vi "popularVideos.vi"(8 "error in (no error)":errorcluster, 11 "ThirdPartyYoutubeLib in":refnum<class "ThirdPartyYoutubeLib.lvclass">) -> (0 "error out":errorcluster, 2 "HashMap":T1, 3 "ThirdPartyYoutubeLib out":refnum<class "ThirdPartyYoutubeLib.lvclass">)   [LabVIEW 2018, in "ThirdPartyYoutubeLib.lvclass"]
uses:
  ThirdPartyYoutubeLib.lvclass
  Globals/HashMap.ctl
  Video Class/Video.lvclass
  ThirdPartyYoutubeLib.lvclass/ThirdPartyYoutubeLib.ctl
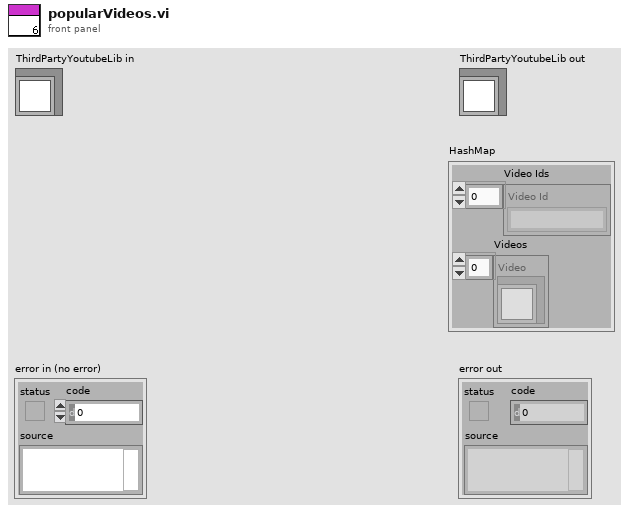
[diagram p1: front panel]
types:
  T1 = typedef "HashMap.ctl" = cluster{"Video Ids":string[], "Videos":refnum<class "Video.lvclass">[]}
  T2 = cluster{"Video Ids":string[], "Videos":refnum<class "Video.lvclass">[]}
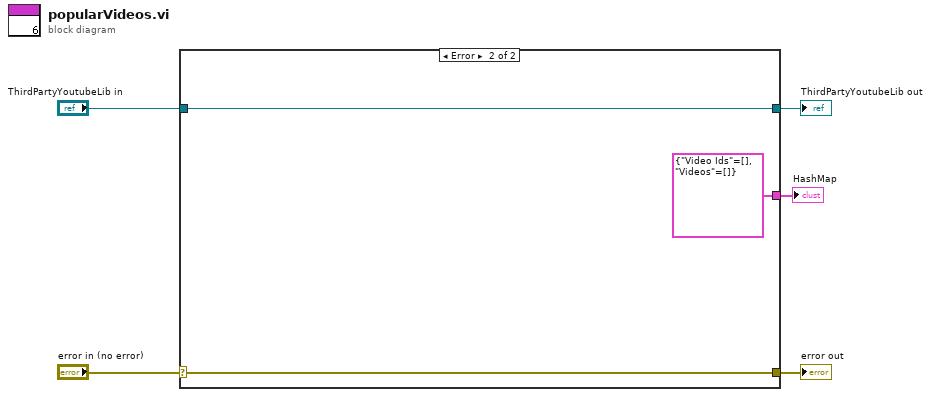
[diagram p0: block diagram]
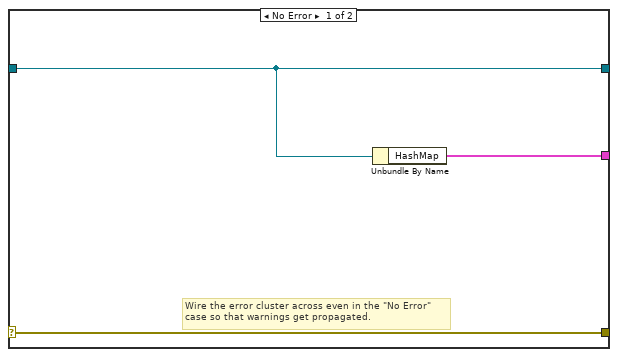
[diagram p2: hidden frame]
diagram:
  n1 = case shown="Error" "error in (no error)" {
    selector: "error in (no error)" -> [w8 w11]
    tunnel: [w8 w11] -> w4
    tunnel: [w7 w10] -> w2
    tunnel: "ThirdPartyYoutubeLib in" -> [w7 w10]
    tunnel: [w6 T2 {"Video Ids"=[], "Videos"=[]} ("HashMap")] -> w1
    frame No Error {
      # "Wire the error cluster across even in the \"No Error\"\ncase so that warnings get propagated."
      n2 = Unbundle By Name(w7) -> ("HashMap"=w6:T2)
    }
    frame Error {
    }
  }
  "error out" <- w4
  "ThirdPartyYoutubeLib out" <- w2
  "HashMap" <- w1
